vi "U3 AIN CR Loop with Chart.vi"() -> ()   [LabVIEW 2021]
panel:
  in  "ms per iteration":i32=500
  in  "stop":bool
  out "Waveform Chart":cluster{"Value Read":dbl, "Value Read":dbl}(graph)
  out "AIN1":dbl format="%.6f"
  out "AIN0":dbl format="%.6f"
  out "Error Message":string
  out "error out":errorcluster
  # "Aquires AIN0 and AIN1 in a loop and adds the readings to a chart each interation."
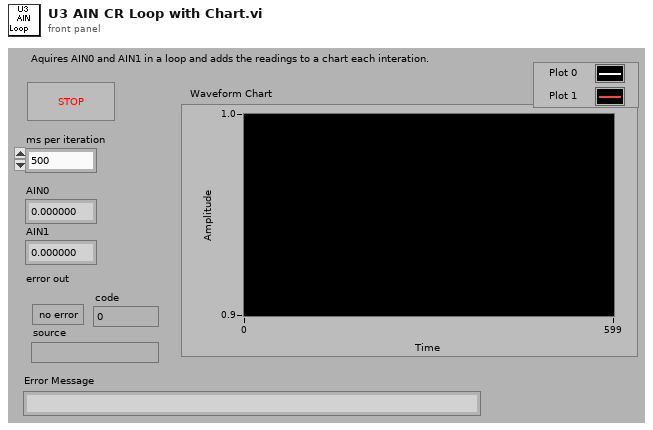
[diagram p1: front panel]
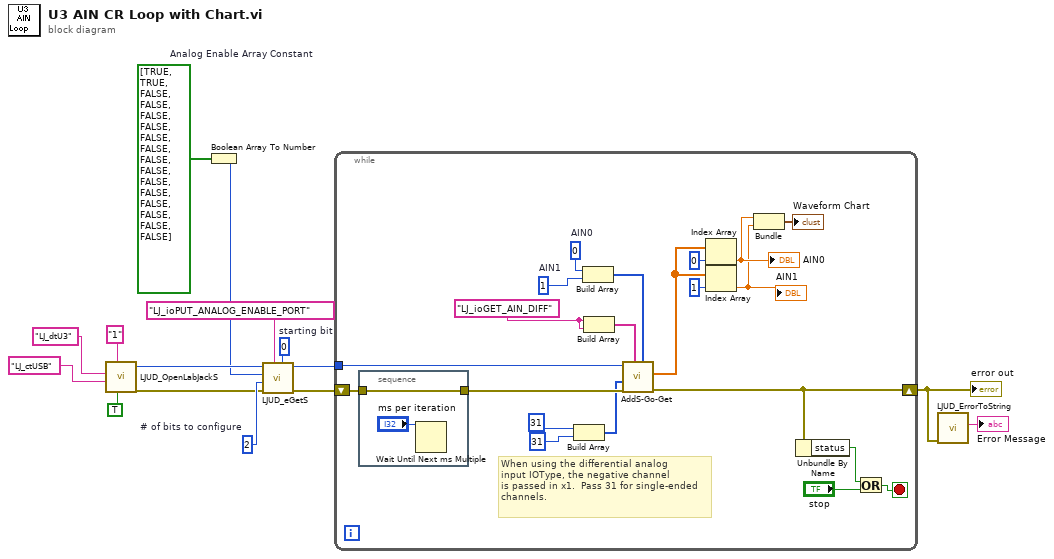
[diagram p0: block diagram]
diagram:
  w6 = 2  # # of bits to configure
  w8 = 0  # starting bit
  w9 = bool[] [TRUE, TRUE, FALSE, FALSE, FALSE, FALSE, FALSE, FALSE, FALSE, FALSE, FALSE, FALSE, FALSE, FALSE, FALSE, FALSE]  # Analog Enable Array Constant
  n1 = call "LJUD_OpenLabJackS.vi"("FirstFound"=TRUE, "Address"="1", "ConnectionType"="LJ_ctUSB", "DeviceType"="LJ_dtU3") -> ("error out"=w4:errorcluster, "Handle"=w5:i32)  [unwired: 5 in, 1 out]
  n2 = Boolean Array To Number(Boolean array=w9) -> (number=w1:u32)
  n3 = call "LJUD_eGetS.vi"("Channel"=w8, "IOType"="LJ_ioPUT_ANALOG_ENABLE_PORT", "error in"=w4, "x1"=w6, "Value Write"=w1, "Handle In"=w5) -> ("error out"=w3:errorcluster, "Handle Out"=w2:i32)  [unwired: 3 in, 1 out]
  n4 = while {
    tunnel: w2 -> [w25]
    shift-left: w3 -> [w22]
    shift-right: [w20] -> w10
    stop <- w24 stop-if-true
    w31 = 1  # AIN1
    w30 = 0  # AIN0
    w32 = "LJ_ioGET_AIN_DIFF" ("IOType")
    # "When using the differential analog\ninput IOType, the negative channel\nis passed in x1.  Pass 31 for single-ended\nchannels."
    n5 = stacked-sequence {
      tunnel: w22 -> [w37]
      tunnel: [w37] -> w21
      frame #0 {
        n6 = Wait Until Next ms Multiple(millisecond multiple="ms per iteration") -> ()  [unwired: 1 out]
      }
    }
    n7 = Build Array(31 ("AIN0"), 31 ("AIN1")) -> (w16:i32[])
    n8 = Build Array(w30, w31) -> (w35:i32[])
    n9 = Build Array(w32, w32) -> (w36:string[])
    n10 = call "AddS-Go-Get.vi"("Channels"=w35, "IOTypes"=w36, "error in"=w21, "x1"=w16, "Handle In"=w25) -> ("error out"=w20:errorcluster, "Values Read"=w29:dbl[])  [unwired: 4 in, 1 out]
    n11 = Index Array(array=w29, index=0 ("Index")) -> (element=w28:dbl)
    "AIN0" <- w28
    n12 = Index Array(array=w29, index=1 ("Index")) -> (element=w27:dbl)
    "AIN1" <- w27
    n13 = Bundle("Value Read"=w28, "Value Read"=w27) -> (→"Waveform Chart":cluster{"Value Read":dbl, "Value Read":dbl})  [unwired: 1 in]
    n14 = Unbundle By Name(w20) -> ("status"=w19:bool)
    n15 = Or(x=w19, y="stop") -> (x .or. y?=w24:bool)
  }
  "error out" <- w10
  n16 = call "LJUD_ErrorToString.vi"("error in"=w10) -> ("String"=→"Error Message":string)  [unwired: 10 in]
